vi "hw2-5 topVI.vi"() -> ()   [LabVIEW 2014]
panel:
  out "Board":bool[][][](array[boolean])
  out "How many solutions":i32
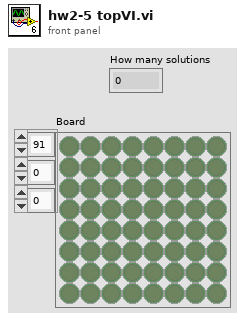
[diagram p1: front panel]
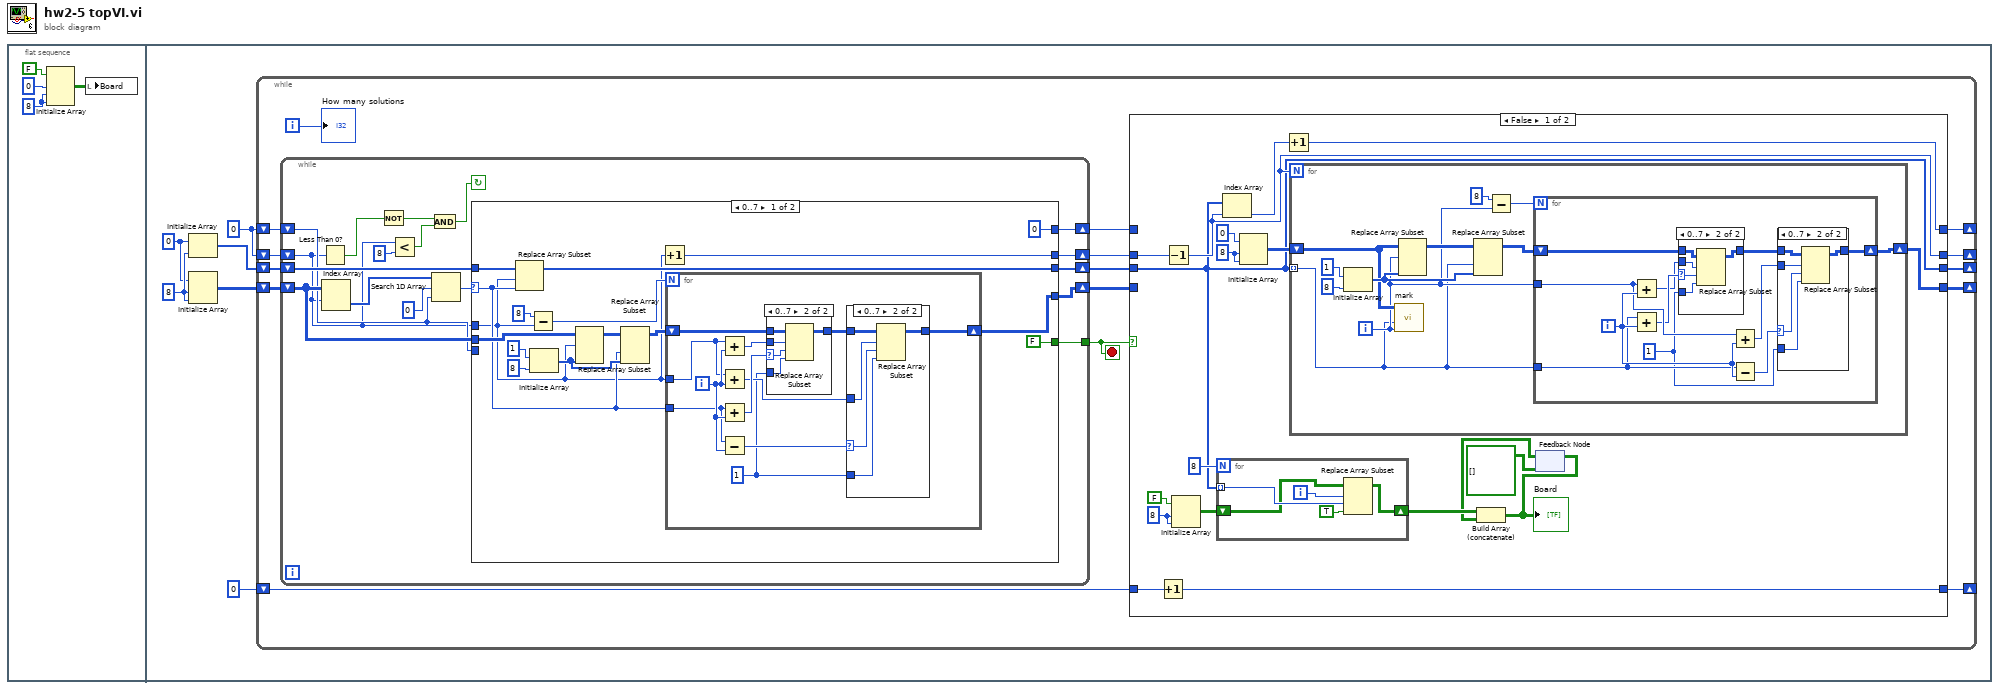
[diagram p0: block diagram]
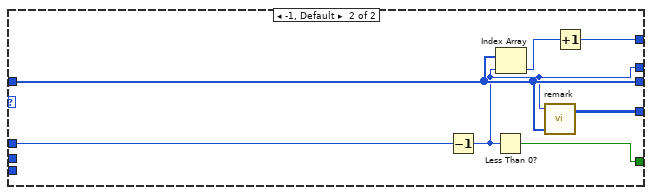
[diagram p7: hidden frame]
diagram:
  n1 = flat-sequence {
    frame #0 {
      w4 = 8 ("dimension size")
      n2 = Initialize Array(FALSE, 0 ("dimension size"), w4, w4) -> (w2:bool[][][])
      n3 = local write "Board"(w2) -> ()
    }
    frame #1 {
      w6 = 0
      w10 = 8
      w9 = 0
      n4 = Initialize Array(w9, w10) -> (w7:i32[])
      n5 = Initialize Array(w9, w10, w10) -> (w8:i32[][])
      n6 = while {
        shift-right: [w15] -> _
        shift-left: w7 -> [w26]
        shift-right: [w14] -> _
        shift-left: w8 -> [w25]
        shift-right: [w13] -> _
        shift-left: w6 -> [w24]
        shift-right: [w12] -> _
        shift-left: w6 -> [w23]
        shift-right: [w16] -> _
        shift-left: 0 -> [w17]
        i -> [w11]
        stop <- w18 stop-if-true
        n7 = while {
          shift-right: [w96] -> w22
          shift-left: w26 -> [w106]
          shift-right: [w97] -> w21
          shift-left: w25 -> [w93]
          shift-right: [w98] -> w20
          shift-left: w24 -> [w92]
          shift-right: [w99] -> w19
          shift-left: w23 -> [w91]
          tunnel: [w100] -> w18
          stop <- w101 continue-if-true
          n8 = Less Than 0?(x=w91) -> (x < 0?=w104:bool)
          n9 = Index Array(array=w93, index (row)=w91) -> (element=w94:i32[])  [unwired: 1 in]
          n10 = Not(x=w104) -> (.not. x?=w103:bool)
          n11 = Less?(x=w91, y=8) -> (x < y?=w102:bool)
          n12 = And(x=w103, y=w102) -> (x .and. y?=w101:bool)
          n13 = Search 1D Array(1D array=w94, element=0, start index (0)=w92) -> (index of element=w90:i32)
          n14 = case shown="0..7" w90 {
            selector: w90 -> [w108 _]
            tunnel: w93 -> [w109 _]
            tunnel: w92 -> [_ _]
            tunnel: w91 -> [w107 w150]
            tunnel: w106 -> [w122 w151]
            tunnel: [w118 w151] -> w96
            tunnel: [w110 w152] -> w97
            tunnel: [w121 w147] -> w99
            tunnel: [0 w148] -> w98
            tunnel: [FALSE w146] -> w100
            frame 0..7 {
              n15 = Replace Array Subset(array=w122, new element=w108, index=w107) -> (w118:i32[])
              n16 = Subtract(x=8, y=w107) -> (x-y=w112:i32)
              n17 = Initialize Array(1 ("element"), 8 ("dimension size")) -> (w115:i32[])
              n18 = Replace Array Subset(array=w109, new element=w115, index (row)=w107) -> (w114:i32[][])  [unwired: 1 in]
              n19 = Replace Array Subset(array=w114, new element=w115, index (col)=w108) -> (w113:i32[][])  [unwired: 1 in]
              n20 = Increment(x=w107) -> (x+1=w121:i32)
              n21 = for {
                N: w112 -> [_]
                tunnel: w107 -> [w128]
                tunnel: w108 -> [w129]
                shift-right: [w131] -> w110
                shift-left: w113 -> [w133]
                i -> [w130]
                w123 = 1
                n22 = Add(x=w128, y=w130) -> (x+y=w125:i32)
                n23 = Add(x=w128, y=w130) -> (x+y=w124:i32)
                n24 = Add(x=w129, y=w130) -> (x+y=w127:i32)
                n25 = Subtract(x=w129, y=w130) -> (x-y=w126:i32)
                n26 = case shown="0..7" w127 {
                  selector: w127 -> [_ w141]
                  tunnel: w133 -> [w140 w145]
                  tunnel: [w140 w144] -> w132
                  tunnel: w125 -> [_ w143]
                  tunnel: w123 -> [_ w142]
                  frame Default {
                  }
                  frame 0..7 {
                    n27 = Replace Array Subset(array=w145, new element=w142, index (row)=w143, index (col)=w141) -> (w144:i32[][])
                  }
                }
                n28 = case shown="0..7" w126 {
                  selector: w126 -> [_ w136]
                  tunnel: w132 -> [w134 w139]
                  tunnel: [w134 w138] -> w131
                  tunnel: w124 -> [_ w137]
                  tunnel: w123 -> [_ w135]
                  frame Default {
                  }
                  frame 0..7 {
                    n29 = Replace Array Subset(array=w139, new element=w135, index (row)=w137, index (col)=w136) -> (w138:i32[][])
                  }
                }
              }
            }
            frame -1, Default {
              n30 = Decrement(x=w150) -> (x-1=w147:i32)
              n31 = Less Than 0?(x=w147) -> (x < 0?=w146:bool)
              n32 = Index Array(array=w151, index=w147) -> (element=w149:i32)
              n33 = call "remark.vi"("ST"=w151, "Y"=w147) -> ("Q_out"=w152:i32[][])  [unwired: 2 in]
              n34 = Increment(x=w149) -> (x+1=w148:i32)
            }
          }
        }
        n35 = case shown="False" w18 {
          tunnel: w22 -> [w27 w88]
          tunnel: w21 -> [_ w87]
          tunnel: w20 -> [_ w86]
          tunnel: w19 -> [w43 w85]
          tunnel: w17 -> [w45 w89]
          tunnel: [w44 w89] -> w16
          tunnel: [w27 w88] -> w15
          tunnel: [w29 w87] -> w14
          tunnel: [w41 w86] -> w13
          tunnel: [w28 w85] -> w12
          frame False {
            w30 = 8 ("dimension size")
            w40 = 8 ("dimension size")
            n36 = Increment(x=w45) -> (x+1=w44:i32)
            n37 = Decrement(x=w43) -> (x-1=w28:i32)
            n38 = Initialize Array(FALSE, w40, w40) -> (w38:bool[][])
            n39 = for {
              N: 8 -> [_]
              tunnel: w27 -> [w84] mode=indexing
              shift-right: [w80] -> w36
              shift-left: w38 -> [w81]
              i -> [w83]
              n40 = Replace Array Subset(array=w81, new element=TRUE, index (row)=w83, index (col)=w84) -> (w80:bool[][])
            }
            n41 = Index Array(array=w27, index=w28) -> (element=w42:i32)
            n42 = Initialize Array(0 ("element"), w30, w30) -> (w32:i32[][])
            n43 = Increment(x=w42) -> (x+1=w41:i32)
            n44 = for {
              N: w28 -> [_]
              shift-right: [w49] -> w29
              shift-left: w32 -> [w48]
              tunnel: w27 -> [w46] mode=indexing
              i -> [w47]
              n45 = Initialize Array(1 ("element"), 8 ("dimension size")) -> (w54:i32[])
              n46 = call "mark.vi"("Y"=w47, "X"=w46, "Q_in"=w48) -> ()  [unwired: 3 in, 1 out]
              n47 = Replace Array Subset(array=w48, new element=w54, index (row)=w47) -> (w53:i32[][])  [unwired: 1 in]
              n48 = Replace Array Subset(array=w53, new element=w54, index (col)=w46) -> (w52:i32[][])  [unwired: 1 in]
              n49 = Subtract(x=8, y=w47) -> (x-y=w51:i32)
              n50 = for {
                N: w51 -> [_]
                tunnel: w47 -> [w62]
                tunnel: w46 -> [w63]
                shift-right: [w65] -> w49
                shift-left: w52 -> [w67]
                i -> [w64]
                w57 = 1
                n51 = Add(x=w62, y=w64) -> (x+y=w59:i32)
                n52 = Add(x=w63, y=w64) -> (x+y=w61:i32)
                n53 = case shown="0..7" w61 {
                  selector: w61 -> [_ w75]
                  tunnel: w67 -> [w74 w79]
                  tunnel: [w74 w78] -> w66
                  tunnel: w59 -> [_ w77]
                  tunnel: w57 -> [_ w76]
                  frame Default {
                  }
                  frame 0..7 {
                    n54 = Replace Array Subset(array=w79, new element=w76, index (row)=w77, index (col)=w75) -> (w78:i32[][])
                  }
                }
                n55 = Add(x=w62, y=w64) -> (x+y=w58:i32)
                n56 = Subtract(x=w63, y=w64) -> (x-y=w60:i32)
                n57 = case shown="0..7" w60 {
                  selector: w60 -> [_ w70]
                  tunnel: w66 -> [w68 w73]
                  tunnel: [w68 w72] -> w65
                  tunnel: w58 -> [_ w71]
                  tunnel: w57 -> [_ w69]
                  frame Default {
                  }
                  frame 0..7 {
                    n58 = Replace Array Subset(array=w73, new element=w69, index (row)=w71, index (col)=w70) -> (w72:i32[][])
                  }
                }
              }
            }
            n59 = feedback #1(bool[][][] []) -> (w35:bool[][][])
            n60 = Build Array (concatenate)(w36, w35) -> (w34:bool[][][])
            "Board" <- w34
            n61 = feedback-in #1(w34) -> ()
          }
          frame True {
          }
        }
        "How many solutions" <- w11
      }
    }
  }
